vi "Test - Serial Device - Write Port 1.vi"(8 "error in (no error)":errorcluster, 11 "Module ID":i32) -> (0 "error out":errorcluster, 3 "Pass":bool)   [LabVIEW 2020]
doc: "_____\nCreated using Delacor QMH Event Scripter 5.0.0.112."
uses:
  Libraries/Serial Device/Serial Device.lvlib
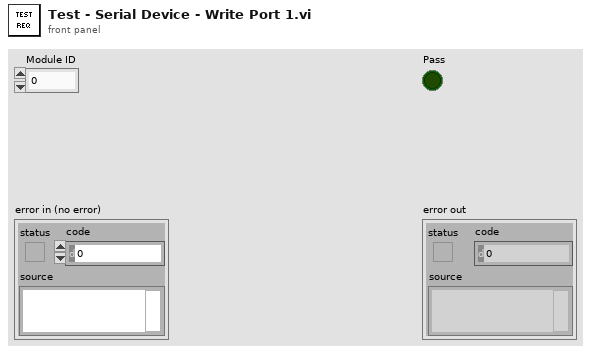
[diagram p1: front panel]
types:
  T1 = typedef "Serial Device.lvlib/Broadcast Events--cluster.ctl" = cluster{"Module Did Init":refnum<user-event>, "Status Updated":refnum<user-event>, "Error Reported":refnum<user-event>, "Module Did Stop":refnum<user-event>, "Update Module Execution Status":refnum<user-event>}
  T2 = typedef "Serial Device.lvlib/Write Port (Reply Payload)--cluster.ctl" = cluster{"Write Port_error":errorcluster, "Response":string}
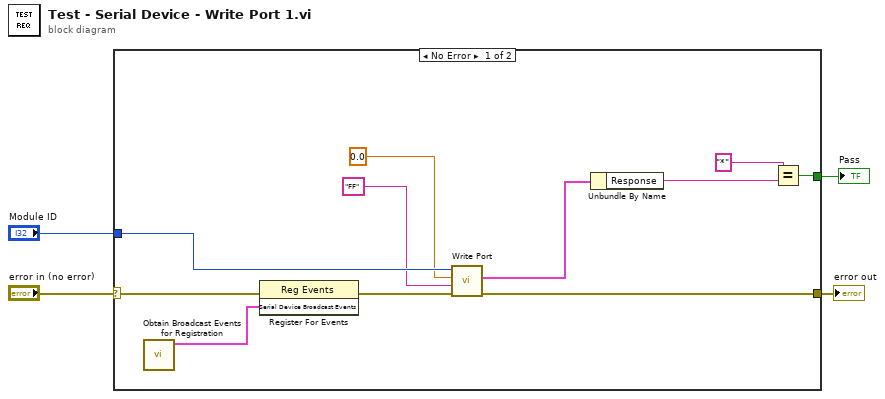
[diagram p0: block diagram]
diagram:
  n1 = case shown="No Error" "error in (no error)" {
    selector: "error in (no error)" -> [w15 w16]
    tunnel: [w9 w16] -> w3
    tunnel: "Module ID" -> [w14 _]
    tunnel: [w8 _] -> w1
    frame No Error {
      n2 = call "Obtain Broadcast Events for Registration.vi"() -> ("Serial Device Broadcast Events"=w12:T1)  [unwired: 9 in, 2 out]
      n3 = register-events(error in=w15, w12) -> (error out=w13:errorcluster)  [unwired: 1 in, 1 out]
      n4 = call "Write Port.vi"("error in (no error)"=w13, "VAL"="FF", "PORT"=0.0, "Module ID"=w14) -> ("error out"=w9:errorcluster, "Reply Payload"=w6:T2)  [unwired: 5 in, 1 out]
      n5 = Unbundle By Name(w6) -> ("Response"=w5:string)
      n6 = Equal?(x="*" ("String"), y=w5) -> (x = y?=w8:bool)
    }
    frame Error {
    }
  }
  "error out" <- w3
  "Pass" <- w1
